vi "request.vi"(0 "Device In":T1, 3 "error in":errorcluster) -> (7 "Device Out":T1, 8 "Comm":T2, 9 "body":string, 10 "error out":errorcluster)   [LabVIEW 2019]
uses:
  <userlib>/IoT Devices/_subVIs/HTTPComm.ctl
  <userlib>/Onshape/_SubVI/Cluster.ctl
  <vilib>/httpClient/POSTBuffer.vi
  <vilib>/httpClient/LabVIEWHTTPClient.lvlib
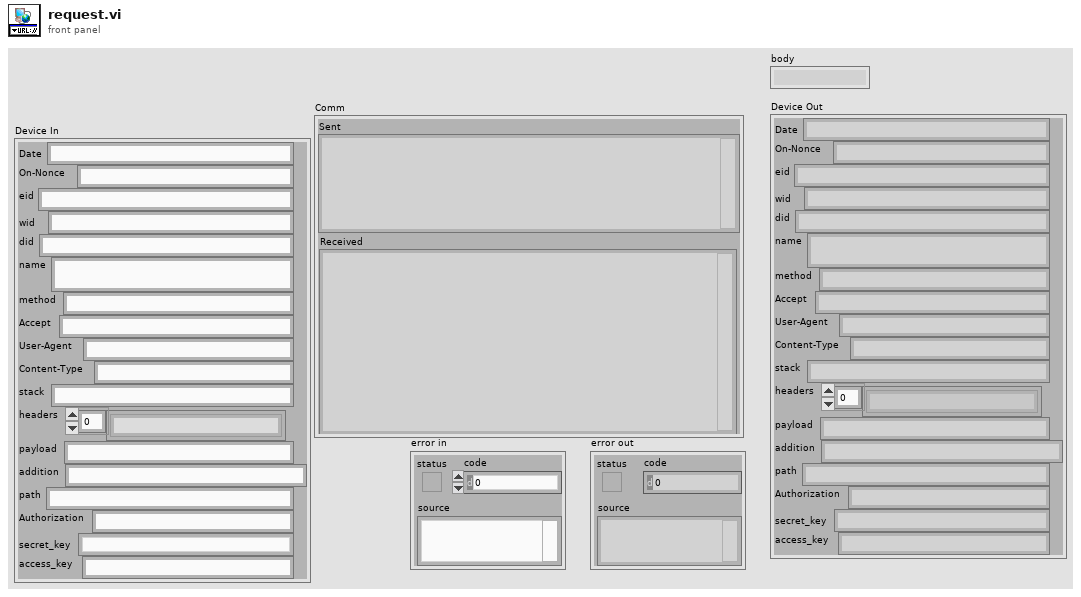
[diagram p1: front panel]
types:
  T1 = typedef "Cluster.ctl" = cluster{"Date":string, "On-Nonce":string, "eid":string, "wid":string, "did":string, "name":string, "method":string, "Accept":string, "User-Agent":string, "Content-Type":string, "stack":string, "headers":string[], "payload":string, "addition":string, "path":string, "Authorization":string, "secret_key":string, "access_key":string}
  T2 = typedef "HTTPComm.ctl" = cluster{"url":string, "sent headers":string, "sent body":string, "headers":string, "body":string, "Sent":string, "Received":string}
  T3 = typedef "LabVIEWHTTPClient.lvlib/ClientHandle.ctl" = refnum<k1>
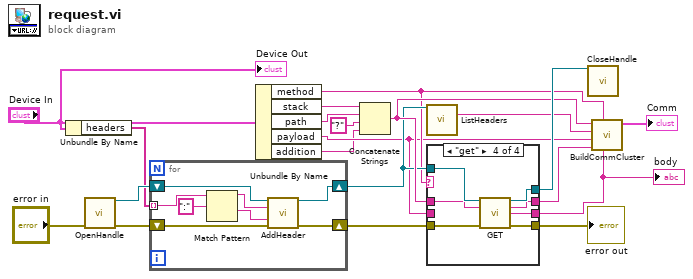
[diagram p0: block diagram]
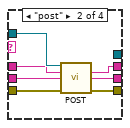
[diagram p3: hidden frame]
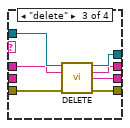
[diagram p4: hidden frame]
diagram:
  n1 = Unbundle By Name("Device In") -> ("headers"=w18:string[])
  n2 = call <vilib>:"OpenHandle.vi"("error in (no error)"="error in") -> ("client handle out"=w19:T3, "error out"=w17:errorcluster)  [unwired: 13 in]
  n3 = for {
    shift-right: [w27] -> w9
    shift-left: w19 -> [w28]
    shift-right: [w25] -> w16
    shift-left: w17 -> [w26]
    tunnel: w18 -> [w21] mode=indexing
    n4 = Match Pattern(string=w21, regular expression=":") -> (before substring=w23:string, after substring=w22:string)  [unwired: 1 in, 2 out]
    n5 = call <vilib>:"AddHeader.vi"("client handle"=w28, "header"=w23, "value"=w22, "error in (no error)"=w26) -> ("client handle out"=w27:T3, "error out"=w25:errorcluster)  [unwired: 10 in]
  }
  n6 = Unbundle By Name("Device In") -> ("method"=w5:string, "stack"=w13:string, "path"=w12:string, "payload"=w4:string, "addition"=w1:string)
  n7 = Concatenate Strings(w13, w12, "?", w1) -> (w10:string)
  n8 = call <vilib>:"ListHeaders.vi"("client handle"=w9) -> ("headers"=w8:string)  [unwired: 12 in, 2 out]
  n9 = case shown="\"get\"" w5 {
    tunnel: w9 -> [_ w36 w43 w50]
    tunnel: [_ _ w42 w49] -> w20
    tunnel: [_ w35 w40 w47] -> w6
    tunnel: [_ w34 w41 w48] -> w7
    tunnel: w16 -> [w29 w33 w39 w46]
    tunnel: [w29 w32 w38 w45] -> w15
    tunnel: w10 -> [_ w31 w37 w44]
    tunnel: w4 -> [_ w30 _ _]
    frame "False", Default {
    }
    frame "post" {
      n10 = call-poly <vilib>:"POST.vi"("client handle"=w36, "url"=w31, "buffer"=w30, "error in (no error)"=w33) -> ("headers"=w34:string, "body"=w35:string, "error out"=w32:errorcluster)  [unwired: 8 in, 1 out]
    }
    frame "delete" {
      n11 = call <vilib>:"DELETE.vi"("client handle"=w43, "url"=w37, "error in (no error)"=w39) -> ("client handle out"=w42:T3, "headers"=w41:string, "body"=w40:string, "error out"=w38:errorcluster)  [unwired: 9 in]
    }
    frame "get" {
      n12 = call <vilib>:"GET.vi"("client handle"=w50, "url"=w44, "error in (no error)"=w46) -> ("client handle out"=w49:T3, "headers"=w48:string, "body"=w47:string, "error out"=w45:errorcluster)  [unwired: 9 in]
    }
  }
  "error out" <- w15
  "body" <- w6
  n13 = call <vilib>:"CloseHandle.vi"("client handle"=w20) -> ()  [unwired: 14 in, 1 out]
  n14 = call <userlib>:"BuildCommCluster.vi"("reply body"=w6, "Type"=w5, "reply headers"=w7, "sent body"=w4, "sent headers"=w8, "url"=w10) -> ("Comm"=→"Comm":T2)  [unwired: 5 in]
  "Device Out" <- "Device In"
